vi "Load Module.vi"(8 "error in (no error)":errorcluster) -> (0 "error out":errorcluster)   [LabVIEW 2020, in "ActorModule.lvlib"]
doc: "This a wrapper VI for the Start Module.vi. By stripping the module-specific controls from its terminals and facilitating a default connector pane, it enables the startup.vi to start this module dynamically (without static linking).\n\n____\nHAMPEL SOFTWARE ENGINEERING v2.6.0 (2023-12-19 10:54)"
uses:
  ActorModule.lvlib
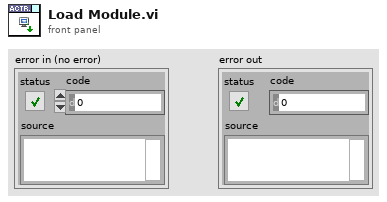
[diagram p1: front panel]
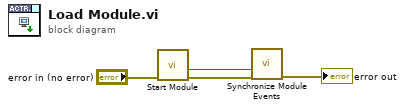
[diagram p0: block diagram]
diagram:
  n1 = call "Start Module.vi"("error in (no error)"="error in (no error)") -> ("error out"=w4:errorcluster, "Wait for Event Sync?"=w1:bool)  [unwired: 7 in, 2 out]
  n2 = call "Synchronize Module Events.vi"("error in (no error)"=w4, "Wait for Event Sync?"=w1) -> ("error out"=→"error out":errorcluster)  [unwired: 9 in]
